vi "MGI Round Up to Power of Two.vi"(1 "Integer":i32) -> (0 "Power of 2 Integer":i32)   [LabVIEW 2016]
doc: "Round up to a power of two.\n\nAuthored by David A Moore\nsupport@mooregoodideas.com\nwww.mooregoodideas.com\n\nCopyright (c) 2010, Moore Good Ideas, Inc.\n\nAll rights reserved.\n\nRedistribution and use in source and binary forms, with or without modification, are permitted provided that the following conditions are met:\n\n * Redistributions of source code must retain the above copyright notice, this list of conditions and the following disclaimer.\n * Redistributions in binary form must reproduce the above copyright notice, this list of conditions and the following disclaimer in the documentation and/or other materials provided with the distribution.\n * Neither the name of Moore Good Ideas, Inc. nor the names of its contributors may be used to endorse or promote products derived from this software without specific prior written permission.\n\nTHIS SOFTWARE IS PROVIDED BY THE COPYRIGHT HOLDERS AND CONTRIBUTORS \"AS IS\" AND ANY EXPRESS OR IMPLIED WARRANTIES, INCLUDING, BUT NOT LIMITED TO, THE IMPLIED WARRANTIES OF MERCHANTABILITY AND FITNESS FOR A PARTICULAR PURPOSE ARE DISCLAIMED. IN NO EVENT SHALL THE COPYRIGHT OWNER OR CONTRIBUTORS BE LIABLE FOR ANY DIRECT, INDIRECT, INCIDENTAL, SPECIAL, EXEMPLARY, OR CONSEQUENTIAL DAMAGES (INCLUDING, BUT NOT LIMITED TO, PROCUREMENT OF SUBSTITUTE GOODS OR SERVICES; LOSS OF USE, DATA, OR PROFITS; OR BUSINESS INTERRUPTION) HOWEVER CAUSED AND ON ANY THEORY OF LIABILITY, WHETHER IN CONTRACT, STRICT LIABILITY, OR TORT (INCLUDING NEGLIGENCE OR OTHERWISE) ARISING IN ANY WAY OUT OF THE USE OF THIS SOFTWARE, EVEN IF ADVISED OF THE POSSIBILITY OF SUCH DAMAGE."
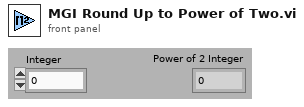
[diagram p1: front panel]
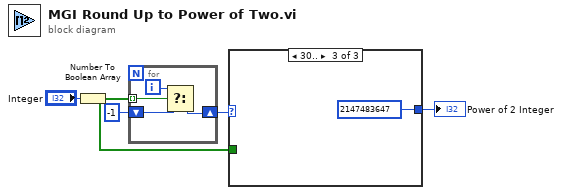
[diagram p0: block diagram]
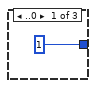
[diagram p2: hidden frame]
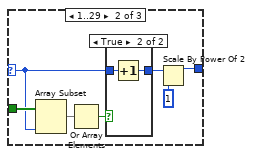
[diagram p3: hidden frame]
diagram:
  n1 = Number To Boolean Array(number="Integer") -> (Boolean array=w4:bool[])
  n2 = for {
    tunnel: w4 -> [w9] mode=indexing
    shift-right: [w6] -> w2
    shift-left: -1 -> [w7]
    i -> [w8]
    n3 = Select(t=w8, s=w9, f=w7) -> (s? t:f=w6:i32)
  }
  n4 = case shown="30.." w2 {
    selector: w2 -> [_ w14 _]
    tunnel: w4 -> [_ w17 _]
    tunnel: [1 ("Power of 2 Integer") w11 2147483647 ("Power of 2 Integer")] -> w1
    frame ..0 {
    }
    frame 1..29 {
      n5 = Array Subset(array=w17, length=w14) -> (w16:bool[])  [unwired: 1 in]
      n6 = Or Array Elements(Boolean array=w16) -> (logical OR=w15:bool)
      n7 = case shown="True" w15 {
        tunnel: w14 -> [w18 w20]
        tunnel: [w18 w19] -> w13
        frame False {
        }
        frame True {
          n8 = Increment(x=w20) -> (x+1=w19:i32)
        }
      }
      n9 = Scale By Power Of 2(n=w13, x=1 ("Power of 2 Integer")) -> (x*2^n=w11:i32)
    }
    frame 30.. {
    }
  }
  "Power of 2 Integer" <- w1
